vi "svc_Generate Bins from Range and Intervals.vi"(10 "range":cluster{"minimum":dbl, "maximum":dbl}={"minimum"=-10.0, "maximum"=10.0}, 11 "number of bins":i32=8) -> (2 "nominal centers":dbl[](array[numeric]), 3 "bins":T1[](array[typedef]) {"upper" format="%0.2f"; "lower" format="%0.2f"})   [LabVIEW 2017]
uses:
  <vilib>/addons/_NISVFA/_Shared subVIs/Controls/svc_Bin Specification.ctl
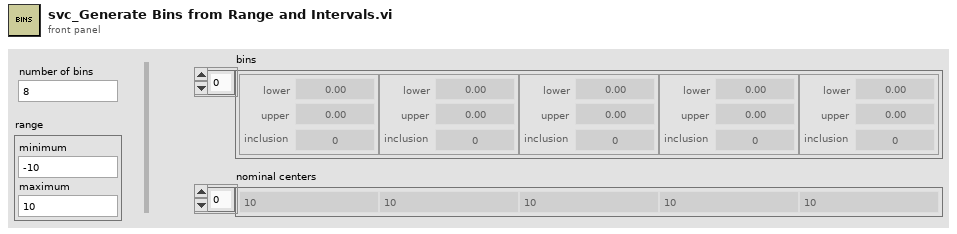
[diagram p1: front panel]
types:
  T1 = typedef "svc_Bin Specification.ctl" = cluster{"lower":dbl, "upper":dbl, "inclusion":u32}
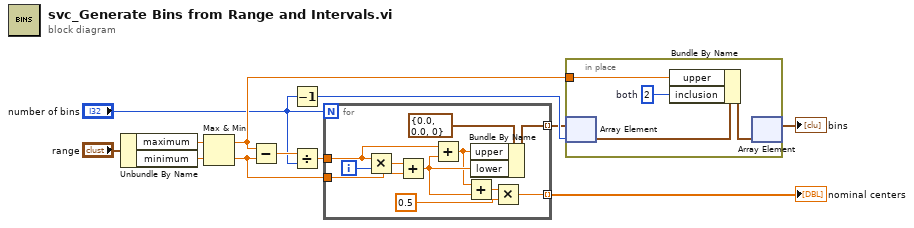
[diagram p0: block diagram]
diagram:
  n1 = Unbundle By Name("range") -> ("maximum"=w2:dbl, "minimum"=w1:dbl)
  n2 = Max & Min(x=w2, y=w1) -> (max(x,y)=w5:dbl, min(x,y)=w11:dbl)
  n3 = Subtract(x=w5, y=w11) -> (x-y=w10:dbl)
  n4 = Decrement(x="number of bins") -> (x-1=w8:i32)
  n5 = Divide(x=w10, y="number of bins") -> (x/y=w9:dbl)
  n6 = for {
    N: "number of bins" -> [_]
    tunnel: [w23] -> w7 mode=indexing
    tunnel: w9 -> [w19]
    tunnel: w11 -> [w21]
    tunnel: [w14] -> w3 mode=indexing
    i -> [w22]
    n7 = Multiply(x=w19, y=w22) -> (x*y=w20:dbl)
    n8 = Add(x=w20, y=w21) -> (x+y=w16:dbl)
    n9 = Add(x=w19, y=w16) -> (x+y=w15:dbl)
    n10 = Add(x=w15, y=w16) -> (x+y=w18:dbl)
    n11 = Bundle By Name(cluster=T1 {"lower"=0.0, "upper"=0.0, "inclusion"=0} ("svc_Bin Specification"), "upper"=w15, "lower"=w16) -> (w23:T1)
    n12 = Multiply(x=w18, y=0.5) -> (x*y=w14:dbl)
  }
  "nominal centers" <- w3
  n13 = in-place {
    in-place-border: w5 -> [w25]
    w24 = u32 2  # both
    n14 = in-place-array #1(w7, w8) -> (w27:T1)
    n15 = Bundle By Name(cluster=w27, "upper"=w25, "inclusion"=w24) -> (w26:T1)
    n16 = in-place-array #1(w26) -> (→"bins":T1[])  [unwired: 1 out]
  }
